vi "Construct RootModelNotifiesWhenStopped.vi"() -> (1 "Final Error Notifier":refnum<notifier>, 3 "RootModelNotifiesWhenStopped out":refnum<class "RootModelNotifiesWhenStopped.lvclass">)   [LabVIEW 2017, in "RootModelNotifiesWhenStopped.lvclass"]
uses:
  RootModelNotifiesWhenStopped.lvclass
  RootModelNotifiesWhenStopped.lvclass/RootModelNotifiesWhenStopped.ctl
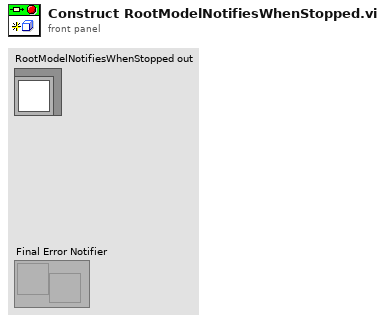
[diagram p1: front panel]
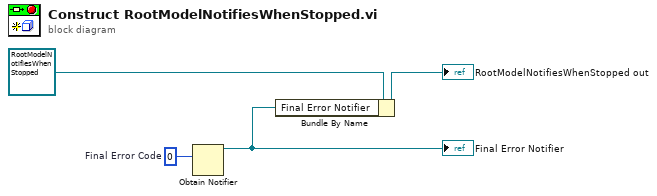
[diagram p0: block diagram]
diagram:
  w3 = 0  # Final Error Code
  n1 = Obtain Notifier(notification data type=w3) -> (notifier out=w1:refnum<notifier>)  [unwired: 3 in, 2 out]
  "Final Error Notifier" <- w1
  n2 = Bundle By Name(cluster=refnum<class "RootModelNotifiesWhenStopped.lvclass"> refnum ("RootModelNotifiesWhenStopped in"), "Final Error Notifier"=w1) -> (→"RootModelNotifiesWhenStopped out":refnum<class "RootModelNotifiesWhenStopped.lvclass">)
